vi "Unary RouteGuide Test.vi"() -> ()   [LabVIEW 2019, in "route_guide_client.lvlib"]
uses:
  route_guide_client.lvlib
  RPC Messages/routeguide_Point.ctl
  RPC Messages/routeguide_Feature.ctl
panel:
  out "error out":errorcluster
  in  "error in":errorcluster
  in  "Server Address":string="localhost:50051"
  out "Response Data":T1
  in  "Request Data":T2={"latitude"=2, "longitude"=2}
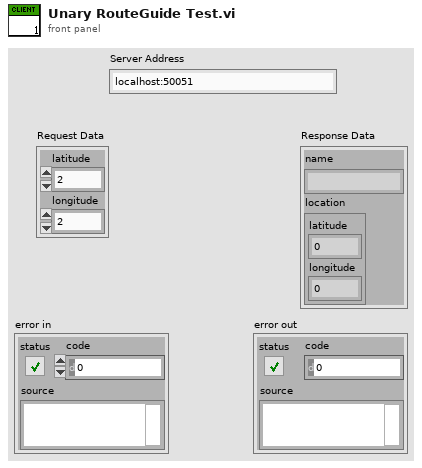
[diagram p1: front panel]
types:
  T1 = typedef "route_guide_client.lvlib/routeguide_Feature.ctl" = cluster{"name":string, "location":T2}
  T2 = typedef "route_guide_client.lvlib/routeguide_Point.ctl" = cluster{"latitude":i32, "longitude":i32}
  T3 = typedef "grpc-lvsupport-release.lvlib/grpcId.ctl" = u64
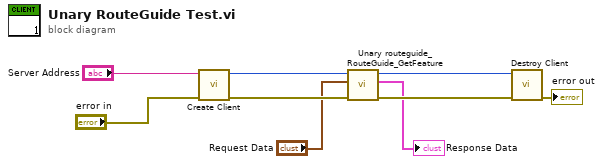
[diagram p0: block diagram]
diagram:
  n1 = call "Create Client.vi"("error in"="error in", "address"="Server Address") -> ("error out"=w8:errorcluster, "gRPC ID Out"=w9:T3)  [unwired: 8 in]
  n2 = call "Unary routeguide_RouteGuide_GetFeature.vi"("error in"=w8, "Request Data"="Request Data", "gRPC ID"=w9) -> ("error out"=w7:errorcluster, "Response Data"=→"Response Data":T1, "gRPC ID out"=w6:T3)  [unwired: 6 in]
  n3 = call "Destroy Client.vi"("error in"=w7, "gRPC ID"=w6) -> ("error out"=→"error out":errorcluster)  [unwired: 9 in]
